vi "test-trajectory-generator-02.vi"() -> (3 "Okay":bool)   [LabVIEW 2019]
uses:
  <vilib>/Rock Robotics/WPI/ThirdParty/JAS_Junk/TrajLib/TRAJECTORY_SPLINE_TYPE_ENUM.ctl
  <vilib>/Rock Robotics/WPI/ThirdParty/JAS_Junk/TrajLib/Translation2d_Create.vi
  <vilib>/Rock Robotics/WPI/ThirdParty/JAS_Junk/TrajLib/Rotation2d_CreateAngle.vi
  <vilib>/Rock Robotics/WPI/ThirdParty/JAS_Junk/TrajLib/Trajectory_Library.lvlib
panel:
  out "TotalTime_Sec":dbl
  out "size(s)":i32
  out "error out":errorcluster
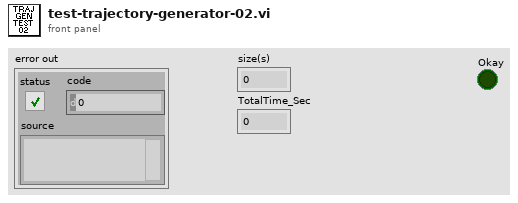
[diagram p1: front panel]
types:
  T1 = typedef "Trajectory_Library.lvlib/TRAJECTORY_SPLINE_TYPE_ENUM.ctl" = enum16{"Cubic", "Cubic With Weights", "Quintic", "Quintic With Weights"}
  T2 = typedef "Trajectory_Library.lvlib/WEIGHTED_WAYPOINT.ctl" = cluster{"TRANSLATION":T3, "ROTATION":T4, "SCALAR":dbl}
  T3 = typedef "Trajectory_Library.lvlib/TRANSLATION2D.ctl" = cluster{"X":dbl, "Y":dbl}
  T4 = typedef "Trajectory_Library.lvlib/ROTATION2D.ctl" = cluster{"VALUE":dbl, "COS":dbl, "SIN":dbl}
  T5 = typedef "Trajectory_Library.lvlib/TRAJ_CONFIG.ctl" = cluster{"MaxVelocity":dbl, "Max Acceleration":dbl, "StartVelocity":dbl, "End Velocity":dbl, "Reversed":bool, "DiffDrKineConstntDefined":bool, "CentAcellConstntDefined":bool, "DiffDrVoltConstntDefined":bool, "DIFF_DRIVE_KINE_CONSTRAINT":T6, "CENTRIPETAL_ACCEL_CONSTRAINT":T8, "SwerveDrKineConstntDefined":bool, "SWERVE_DRIVE_KINE_CONSTRAINT":T9, "DIFF_DRIVE_VOLTAGE_CONSTRAINT":T12, "MECANUM_DRIVE_KINE_CONSTRAINT":T14, "MecanumDrKineConstntDefined":bool}
  T6 = typedef "Trajectory_Library.lvlib/TRAJ_CONSTRAINT_DIIF_DRIVE_KINEMATICS.ctl" = cluster{"Max Speed (M/S)":dbl, "DIFF_DRIVE_KINEMATICS":T7, "Max Accel (M/S2)":dbl}
  T7 = typedef "Trajectory_Library.lvlib/DIFF_DRIVE_KINEMATICS.ctl" = cluster{"TrackWidth_Meters":dbl}
  T8 = typedef "Trajectory_Library.lvlib/TRAJ_CONSTRAINT_CENTRIPETAL_ACCEL.ctl" = cluster{"Max Cent Accel":dbl}
  T9 = typedef "Trajectory_Library.lvlib/TRAJ_CONSTRAINT_SWERVE_DRIVE_KINEMATICS.ctl" = cluster{"Max Speed (M/S)":dbl, "SwerveKinematics":T10}
  T10 = typedef "Trajectory_Library.lvlib/SWERVE_DRIVE_KINEMATICS.ctl" = cluster{"NumModules":i32, "InverseKinematics":T11, "ForwardKinematics":T11, "Modules":T3[], "PrevCoR":T3}
  T11 = typedef "NI_Matrix.lvlib/RealMatrix.ctl" = dbl[][]
  T12 = typedef "Trajectory_Library.lvlib/TRAJ_CONSTRAINT_DIIF_DRIVE_VOLTAGE.ctl" = cluster{"Max Voltage":dbl, "DIFF_DRIVE_KINEMATICS":T7, "SIMPLE_MOTOR_FF":T13}
  T13 = typedef "Trajectory_Library.lvlib/SIMPLE_MOTOR_FF.ctl" = cluster{"Ks":dbl, "Kv":dbl, "Ka":dbl}
  T14 = typedef "Trajectory_Library.lvlib/TRAJ_CONSTRAINT_MECA_DRIVE_KINEMATICS.ctl" = cluster{"Max Speed (M/S)":dbl, "MECA_DRIVE_KINEMATICS":T15}
  T15 = typedef "Trajectory_Library.lvlib/MECA_DRIVE_KINEMATICS.ctl" = cluster{"FrontLeft":T3, "FrontRight":T3, "RearLeft":T3, "RearRight":T3, "InverseKinematics":T11, "ForwardKinematics":T11, "PrevCoR":T3}
  T16 = typedef "Trajectory_Library.lvlib/TRAJECTORY.ctl" = cluster{"TotalTImeSecs":dbl, "States":T17[]}
  T17 = typedef "Trajectory_Library.lvlib/TRAJ_STATE.ctl" = cluster{"TimeSeconds":dbl, "Velocity":dbl, "Acceleration":dbl, "POSE":T18, "Curvature":dbl}
  T18 = typedef "Trajectory_Library.lvlib/POSE2D.ctl" = cluster{"TRANSLATION":T3, "ROTATION":T4}
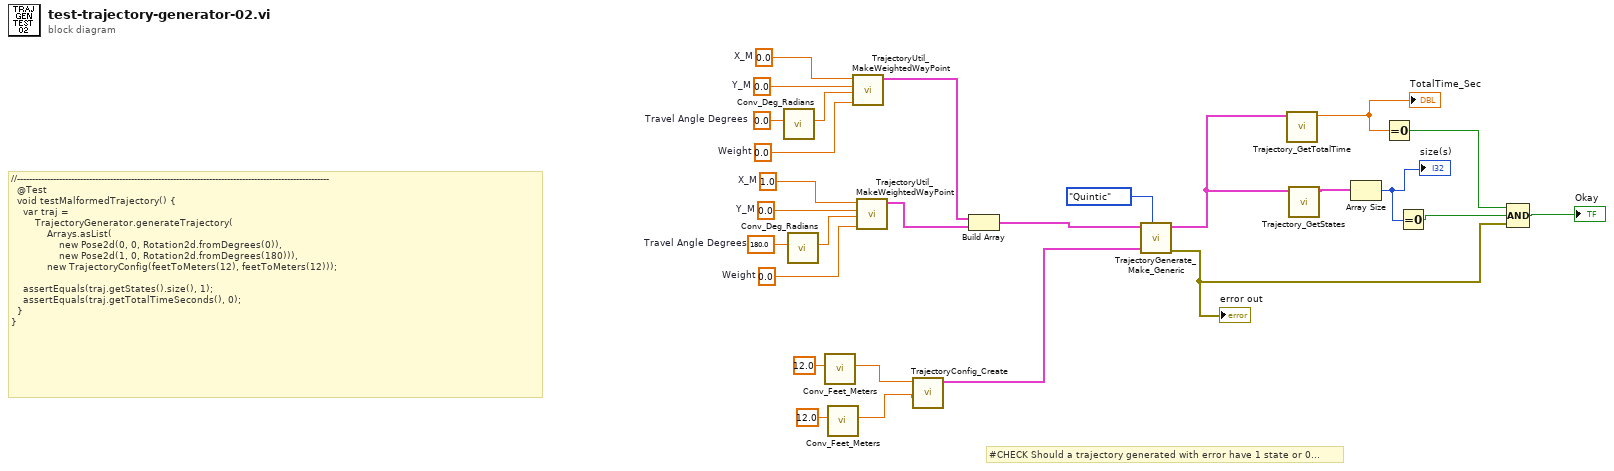
[diagram p0: block diagram]
diagram:
  w24 = 1.0  # X_M
  w23 = 0.0  # Y_M
  w25 = 180.0  # Travel Angle Degrees
  w22 = 0.0  # Weight
  w19 = 0.0  # X_M
  w18 = 0.0  # Y_M
  w20 = 0.0  # Travel Angle Degrees
  w17 = 0.0  # Weight
  # "#CHECK Should a trajectory generated with error have 1 state or 0..."
  # "//--------------------------------------------------------------------------------------------------------\n  @Test\n  void testMalformedTrajectory() {\n    var traj =\n        TrajectoryGenerator.generateTrajectory(\n            Arrays.asList(\n                new Pose2d(0, 0, Rotation2d.fromDegrees(0)),\n                new Pose2d(1, 0, Rotation2d.fromDegrees(180))),\n            new TrajectoryConfig(feetToMeters(12), feetToMeters(12)));\n\n    assertEquals(traj.getStates().size(), 1);\n    assertEquals(traj.getTotalTimeSeconds(), 0);\n  }\n}"
  n1 = call <vilib>:"Conv_Deg_Radians.vi"("Degress"=w20) -> ("Radians"=w21:dbl)  [unwired: 10 in]
  n2 = call <vilib>:"Conv_Deg_Radians.vi"("Degress"=w25) -> ("Radians"=w26:dbl)  [unwired: 10 in]
  n3 = call <vilib>:"Conv_Feet_Meters.vi"("Feet"=12.0) -> ("Meters"=w10:dbl)  [unwired: 10 in]
  n4 = call <vilib>:"Conv_Feet_Meters.vi"("Feet"=12.0) -> ("Meters"=w9:dbl)  [unwired: 10 in]
  n5 = call <vilib>:"TrajectoryUtil_MakeWeightedWayPoint.vi"("Weight"=w17, "Travel Angle Radians"=w21, "Y_M"=w18, "X_M"=w19) -> ("WEIGHTED_WAYPOINT"=w13:T2)  [unwired: 7 in]
  n6 = call <vilib>:"TrajectoryUtil_MakeWeightedWayPoint.vi"("Weight"=w22, "Travel Angle Radians"=w26, "Y_M"=w23, "X_M"=w24) -> ("WEIGHTED_WAYPOINT"=w27:T2)  [unwired: 7 in]
  n7 = call <vilib>:"TrajectoryConfig_Create.vi"("MaxAcceleration"=w9, "MaxVelocity"=w10) -> ("TRAJECTORY_CONFIG"=w16:T5)  [unwired: 9 in]
  n8 = Build Array(w13, w27) -> (w14:T2[])
  n9 = call <vilib>:"TrajectoryGenerate_Make_Generic.vi"("Spline Type"=TRAJECTORY_SPLINE_TYPE_ENUM."Quintic", "traj_config"=w16, "WeightedWayPoints"=w14) -> ("error out"=w6:errorcluster, "TRAJECTORY"=w7:T16)  [unwired: 7 in]
  "error out" <- w6
  n10 = call <vilib>:"Trajectory_GetTotalTime.vi"("TRAJECTORY"=w7) -> ("TotalTime_Sec"=w4:dbl)  [unwired: 10 in]
  "TotalTime_Sec" <- w4
  n11 = call <vilib>:"Trajectory_GetStates.vi"("TRAJECTORY"=w7) -> ("States"=w8:T17[])  [unwired: 10 in]
  n12 = Array Size(array=w8) -> (size(s)=w2:i32)
  "size(s)" <- w2
  n13 = Equal To 0?(x=w4) -> (x = 0?=w3:bool)
  n14 = Equal To 0?(x=w2) -> (x = 0?=w1:bool)
  n15 = Compound Arithmetic op=AND(w3, w1, w6) -> (→"Okay":bool)
